vi "SpectrumWindowExit.vi"() -> ()   [LabVIEW 2012]
panel:
  in  "ExitFlag":bool
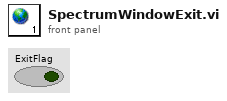
[diagram p1: front panel]
diagram:
